vi "case_load_gcode.vi"(5 "Uninitialized message":string, 7 "initialized":bool, 8 "error in (no error)":errorcluster, 10 "message cluster":T1, 11 "Main VI reference":refnum<vi>) -> (0 "error out":errorcluster)   [LabVIEW 2020]
uses:
  controls/message cluster.ctl
  b4c091be-0a65-48d9-a70c-1f657d6bbbdc.vi
  099df7d6-1651-4c19-8571-9519d06f482d.vi
  feb5f9cc-d726-4795-a7cb-2bed1c3291d7.vi
  f18c196a-35f4-4bf2-ba2e-6796baa24589.vi
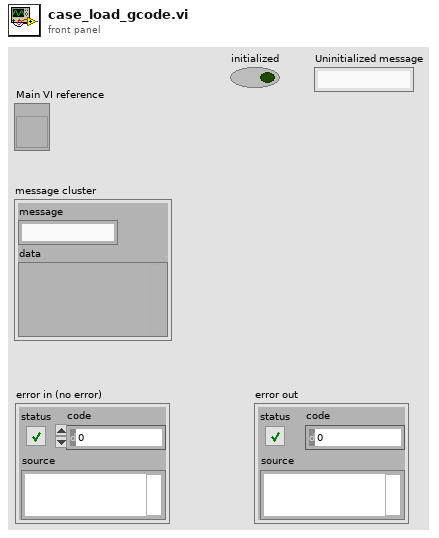
[diagram p1: front panel]
types:
  T1 = typedef "message cluster.ctl" = cluster{"message":string, "data":variant}
  T2 = enum8{"Enabled", "Disabled", "Disabled and Grayed Out"}
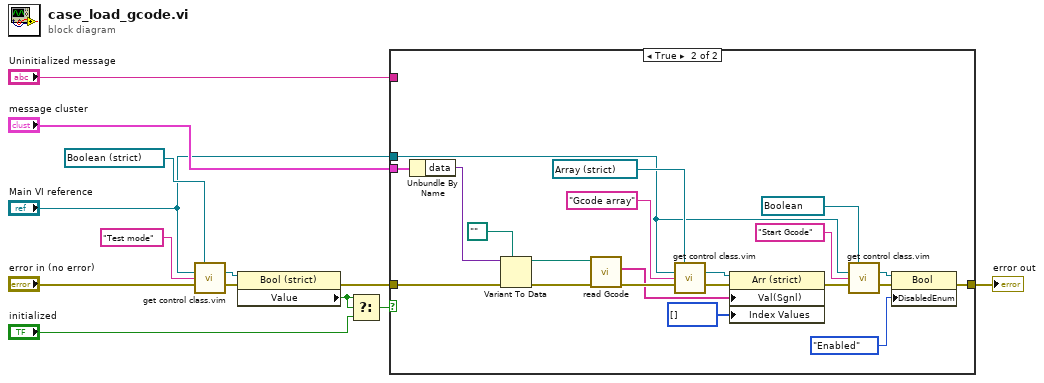
[diagram p0: block diagram]
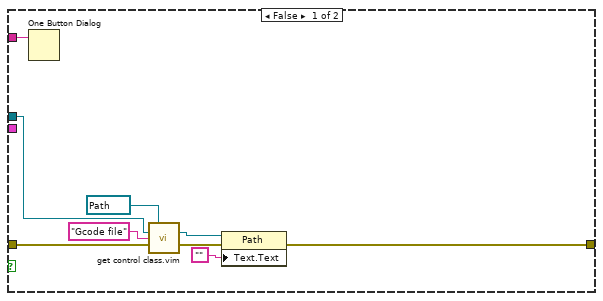
[diagram p2: hidden frame]
diagram:
  n1 = call "get control class.vim"("Control class"=refnum<vi> refnum ("Test mode"), "Main VI reference"="Main VI reference", "Label"="Test mode", "error in (no error)"="error in (no error)") -> ("Control out"=w6:refnum<vi>, "error out"=w5:errorcluster)  [unwired: 10 in]
  n2 = property class="Bool (strict)"(reference=w6, error in=w5) -> (error out=w2:errorcluster, "Value"=w4:bool)  [unwired: 1 out]
  n3 = Select(t=w4, s=w4, f="initialized") -> (s? t:f=w13:bool)
  n4 = case shown="True" w13 {
    tunnel: "message cluster" -> [_ w43]
    tunnel: w2 -> [w17 w38]
    tunnel: [w15 w36] -> w10
    tunnel: "Uninitialized message" -> [w22 _]
    tunnel: "Main VI reference" -> [w14 w24]
    frame False {
      n5 = One Button Dialog(message=w22) -> ()  [unwired: 1 in, 1 out]
      n6 = call "get control class.vim"("Control class"=refnum<vi> refnum ("Gcode file"), "Main VI reference"=w14, "Label"="Gcode file", "error in (no error)"=w17) -> ("Control out"=w18:refnum<vi>, "error out"=w16:errorcluster)  [unwired: 10 in]
      n7 = property on="Property Node" class="Path"(reference=w18, error in=w16, "Text.Text"="") -> (error out=w15:errorcluster)  [unwired: 1 out]
    }
    frame True {
      n8 = Unbundle By Name(w43) -> ("data"=w42:variant)
      n9 = Variant To Data(error in=w38, type=path "", Variant=w42) -> (data=w40:path, error out=w39:errorcluster)
      n10 = call "read Gcode.vi"("error in"=w39, "Gcode path (use dialog)"=w40) -> ("error out"=w32:errorcluster, "Gcode Array"=w23:string[])  [unwired: 7 in, 1 out]
      n11 = call "get control class.vim"("Control class"=refnum<vi> refnum ("Gcode array"), "Main VI reference"=w24, "Label"="Gcode array", "error in (no error)"=w32) -> ("Control out"=w30:refnum<vi>, "error out"=w31:errorcluster)  [unwired: 10 in]
      n12 = property on="Property Node" class="Arr (strict)"(reference=w30, error in=w31, "Val(Sgnl)"=w23, "Index Values"=u32[] []) -> (error out=w27:errorcluster)  [unwired: 1 out]
      n13 = call "get control class.vim"("Control class"=refnum<vi> refnum ("Start Gcode"), "Main VI reference"=w24, "Label"="Start Gcode", "error in (no error)"=w27) -> ("Control out"=w25:refnum<vi>, "error out"=w26:errorcluster)  [unwired: 10 in]
      n14 = property on="Property Node" class="Bool"(reference=w25, error in=w26, "DisabledEnum"=T2."Enabled" ("Disabled")) -> (error out=w36:errorcluster)  [unwired: 1 out]
    }
  }
  "error out" <- w10
